vi "CONEX-ALL Get Controller Version v2.vi"(9 "Expected Device (CONEX-CC)":string="CONEX-CC", 11 "Connection Cluster in":T1) -> (1 "Controller Version":string, 2 "IsExpectedDevice?":bool, 3 "Connection Cluster out":T1, 4 "Response":string)   [LabVIEW 2013]
doc: "VE - Get controller revision information\n\nInput: Expected Device (CONEX-CC) (optional string to check controller name against)\n\nOutput: \nResponse: Raw response string\nController Version: Version returned\nIsExpectedDevice: T/F if Controller Version string contains Expected Device string. This is used to verify the device is what is expected."
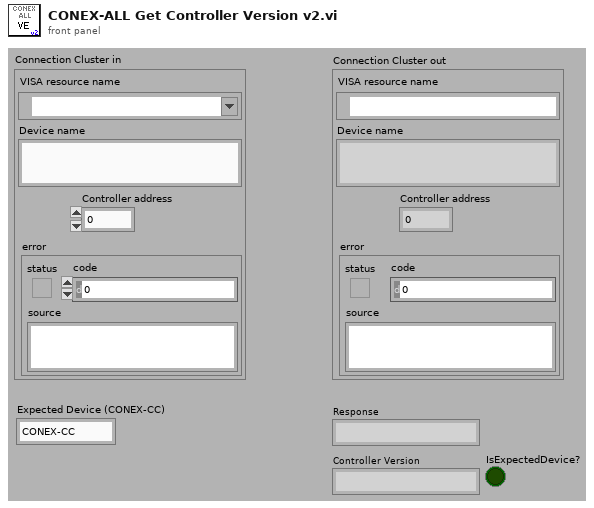
[diagram p1: front panel]
types:
  T1 = cluster{"VISA resource name":refnum<visa-resource-name>, "Device name":string, "Controller address":i32, "error":errorcluster}
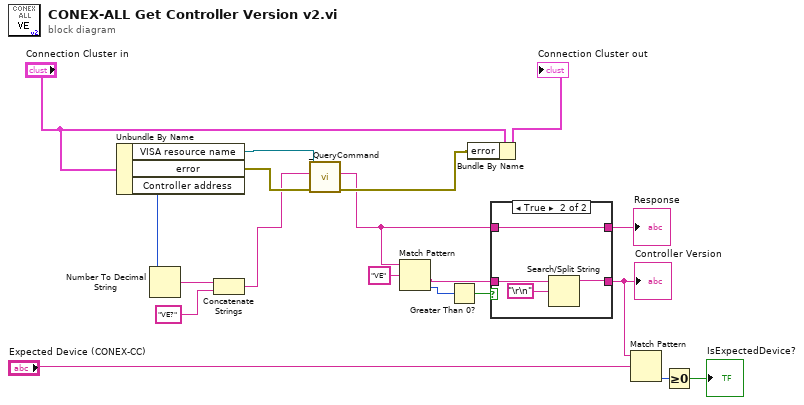
[diagram p0: block diagram]
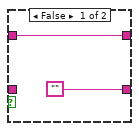
[diagram p2: hidden frame]
diagram:
  n1 = Unbundle By Name("Connection Cluster in") -> ("VISA resource name"=w9:refnum<visa-resource-name>, "error"=w7:errorcluster, "Controller address"=w2:i32)
  n2 = Number To Decimal String(number=w2) -> (decimal integer string=w19:string)  [unwired: 1 out]
  n3 = Concatenate Strings(w19, "VE?" ("strCommand")) -> (w4:string)
  n4 = call "_QueryCommand.vi"("error in"=w7, "Command"=w4, "Instrument Channel in"=w9) -> ("error out"=w8:errorcluster, "Response"=w3:string)  [unwired: 6 in, 1 out]
  n5 = Match Pattern(string=w3, regular expression="VE" ("expression régulière")) -> (after substring=w16:string, offset past match=w15:i32)  [unwired: 3 out]
  n6 = Greater Than 0?(x=w15) -> (x > 0?=w14:bool)
  n7 = Bundle By Name(cluster="Connection Cluster in", "error"=w8) -> (→"Connection Cluster out":T1)
  n8 = case shown="True" w14 {
    tunnel: w3 -> [w21 w25]
    tunnel: w16 -> [_ w23]
    tunnel: [w21 w25] -> w13
    tunnel: ["" w22] -> w11
    frame False {
    }
    frame True {
      n9 = Search/Split String(string=w23, search string/char (-)="\r\n") -> (substring before match=w22:string)  [unwired: 3 out]
    }
  }
  "Response" <- w13
  "Controller Version" <- w11
  n10 = Match Pattern(string=w11, regular expression="Expected Device (CONEX-CC)") -> (offset past match=w12:i32)  [unwired: 4 out]
  n11 = Greater Or Equal To 0?(x=w12) -> (x >= 0?=→"IsExpectedDevice?":bool)
